vi "MeasAction.vi"(8 "error in (no error)":errorcluster caption="entrée d'erreur (pas d'erreur)", 9 "CurvePointIndex":i32, 10 "AllPointIndex":i32, 11 "DefaultDevIn":refnum<class "LeafMagnetometer.lvclass"> caption="DNL_LabVIEW Object in") -> (0 "error out":errorcluster caption="sortie d'erreur", 2 "MeasDatOut":dbl[](array[numeric]), 3 "DefaultDevOut":refnum<class "LeafMagnetometer.lvclass"> caption="DNL_LabVIEW Object out")   [LabVIEW 2012, in "LeafMagnetometer.lvclass"]
uses:
  LeafMagnetometer.lvclass
  LeafMagnetometer.lvclass/LeafMagnetometer.ctl
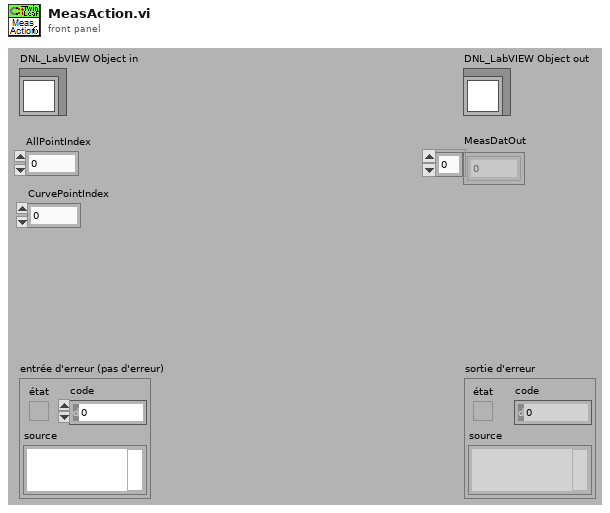
[diagram p1: front panel]
types:
  T1 = typedef "LeafMagnetometer.lvclass/LeafMagnetometer_Func.ctl" = enum16{"Read Fields (nT,nT,nT,nT)", "Read AVM Fields (nT)"}
  T2 = cluster{"Name":string, "Waveform":cluster{"start":dbl, "dt":dbl, "Timeseries":dbl[][]}}[][]
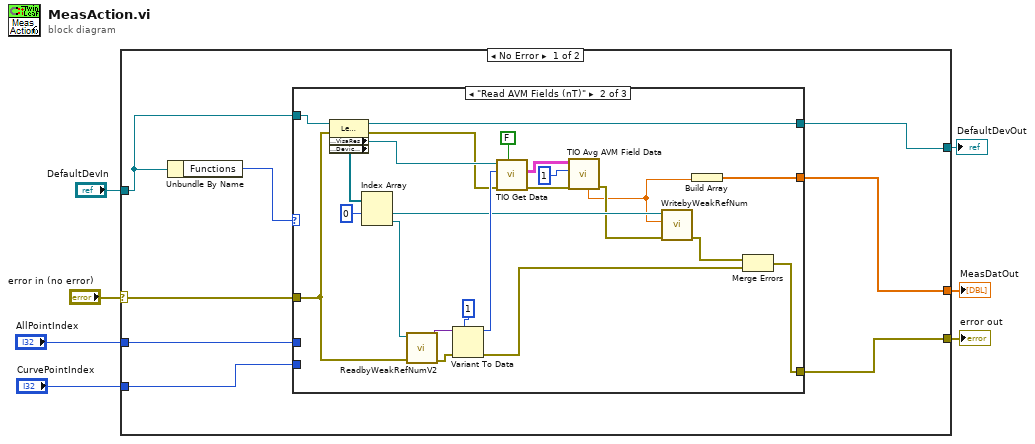
[diagram p0: block diagram]
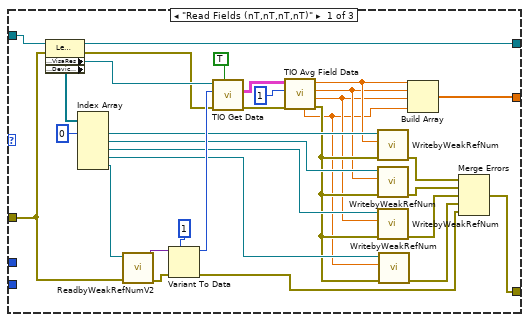
[diagram p2: hidden frame]
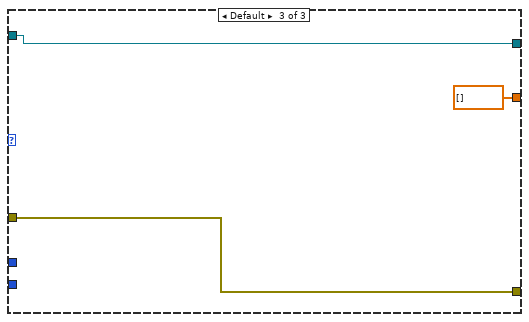
[diagram p3: hidden frame]
diagram:
  n1 = case shown="No Error" "error in (no error)" {
    selector: "error in (no error)" -> [w11 w74]
    tunnel: "DefaultDevIn" -> [w9 w75]
    tunnel: [w8 w75] -> w5
    tunnel: "AllPointIndex" -> [w15 _]
    tunnel: [w14 w74] -> w3
    tunnel: [w13 _] -> w2
    tunnel: "CurvePointIndex" -> [w10 _]
    frame No Error {
      n2 = Unbundle By Name(w9) -> ("Functions"=w12:T1)
      n3 = case shown="\"Read AVM Fields (nT)\"" w12 {
        tunnel: w15 -> [_ _ _]
        tunnel: [w22 w53 w72] -> w14
        tunnel: [w33 w57 dbl[] [] ("Outputs")] -> w13
        tunnel: w11 -> [w36 w59 w72]
        tunnel: w10 -> [_ _ _]
        tunnel: w9 -> [w47 w70 w71]
        tunnel: [w46 w69 w71] -> w8
        frame "Read Fields (nT,nT,nT,nT)" {
          n4 = property class="LeafMagnetometer.lvclass"(reference=w47, error in=w36) -> (reference out=w46:refnum<class "LeafMagnetometer.lvclass">, error out=w35:errorcluster, "Accessor:VisaRes"=w45:refnum<visa-resource-name>, "Accessor:DeviceCtrl"=w41:refnum<vi>[])
          n5 = Index Array(array=w41, index #1=0 ("indice")) -> (element #1=w32:refnum<vi>, element #2=w31:refnum<vi>, element #3=w30:refnum<vi>, element #4=w29:refnum<vi>, element #5=w34:refnum<vi>)  [unwired: 4 in]
          n6 = call <userlib>:"ReadbyWeakRefNumV2.vi"("error in"=w36, "Control Ref"=w34) -> ("error out"=w37:errorcluster, "Valeur"=w39:variant)  [unwired: 8 in]
          n7 = Variant To Data(error in=w37, type=u32 1 ("Samples Count"), Variant=w39) -> (data=w38:u32, error out=w23:errorcluster)
          n8 = call <userlib>:"TIO Get Data.vi"("Type(T:GMR)"=TRUE, "entrée d'erreur (pas d'erreur)"=w35, "Samples Count"=w38, "Nom de ressource VISA"=w45) -> ("sortie d'erreur"=w42:errorcluster, "Tableau"=w44:T2)  [unwired: 5 in, 1 out]
          n9 = call <userlib>:"TIO Avg Field Data.vi"("entrée d'erreur (pas d'erreur)"=w42, "Component Index"=1, "Tableau"=w44) -> ("sortie d'erreur"=w28:errorcluster, "Z Average"=w19:dbl, "Y Average"=w20:dbl, "X Average"=w21:dbl, "Total Average"=w18:dbl)  [unwired: 2 in, 2 out]
          n10 = call <userlib>:"WritebyWeakRefNum.vi"("error in"=w28, "Valeur"=w21, "Control Ref"=w32) -> ("error out"=w27:errorcluster)  [unwired: 8 in]
          n11 = call <userlib>:"WritebyWeakRefNum.vi"("error in"=w28, "Valeur"=w20, "Control Ref"=w31) -> ("error out"=w26:errorcluster)  [unwired: 8 in]
          n12 = call <userlib>:"WritebyWeakRefNum.vi"("error in"=w28, "Valeur"=w19, "Control Ref"=w30) -> ("error out"=w25:errorcluster)  [unwired: 8 in]
          n13 = call <userlib>:"WritebyWeakRefNum.vi"("error in"=w28, "Valeur"=w18, "Control Ref"=w29) -> ("error out"=w24:errorcluster)  [unwired: 8 in]
          n14 = Build Array(w21, w20, w19, w18) -> (w33:dbl[])
          n15 = Merge Errors(w27, w26, w25, w24, w23) -> (w22:errorcluster)
        }
        frame "Read AVM Fields (nT)" {
          n16 = property class="LeafMagnetometer.lvclass"(reference=w70, error in=w59) -> (reference out=w69:refnum<class "LeafMagnetometer.lvclass">, error out=w58:errorcluster, "Accessor:VisaRes"=w68:refnum<visa-resource-name>, "Accessor:DeviceCtrl"=w64:refnum<vi>[])
          n17 = Index Array(array=w64, index #1=0 ("indice")) -> (element #1=w56:refnum<vi>, element #2=w51:refnum<vi>)  [unwired: 1 in]
          n18 = call <userlib>:"ReadbyWeakRefNumV2.vi"("error in"=w59, "Control Ref"=w51) -> ("error out"=w60:errorcluster, "Valeur"=w62:variant)  [unwired: 8 in]
          n19 = Variant To Data(error in=w60, type=u32 1 ("Samples Count"), Variant=w62) -> (data=w61:u32, error out=w50:errorcluster)
          n20 = call <userlib>:"TIO Get Data.vi"("Type(T:GMR)"=FALSE, "entrée d'erreur (pas d'erreur)"=w58, "Samples Count"=w61, "Nom de ressource VISA"=w68) -> ("sortie d'erreur"=w65:errorcluster, "Tableau"=w67:T2)  [unwired: 5 in, 1 out]
          n21 = call <userlib>:"TIO Avg AVM Field Data.vi"("entrée d'erreur (pas d'erreur)"=w65, "Component Index"=1, "Tableau"=w67) -> ("sortie d'erreur"=w55:errorcluster, "Total Average"=w48:dbl)  [unwired: 5 in, 2 out]
          n22 = call <userlib>:"WritebyWeakRefNum.vi"("error in"=w55, "Valeur"=w48, "Control Ref"=w56) -> ("error out"=w54:errorcluster)  [unwired: 8 in]
          n23 = Build Array(w48) -> (w57:dbl[])
          n24 = Merge Errors(w54, w50) -> (w53:errorcluster)
        }
        frame Default {
        }
      }
    }
    frame Error {
    }
  }
  "error out" <- w3
  "DefaultDevOut" <- w5
  "MeasDatOut" <- w2
